vi "Valves_Combination.vi"   [LabVIEW 2011]
uses:
  Pumps_Valves_Dependencies_Global.vi
panel:
  # "Everything is in the block diagram.This vi updates the global combination booleans."
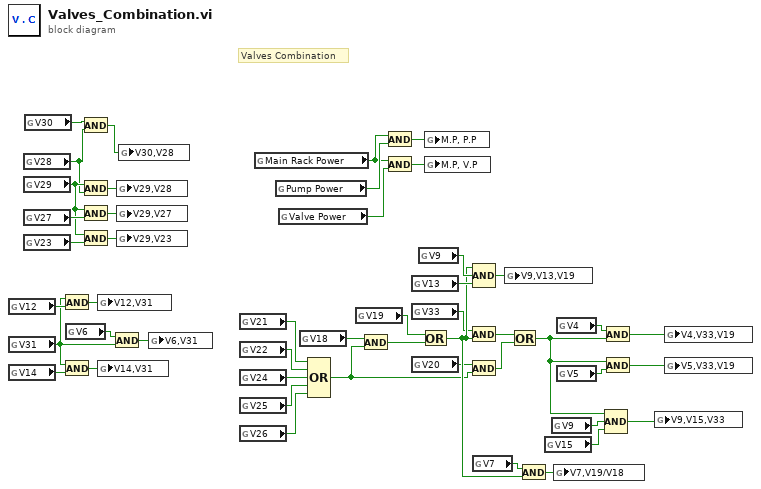
[diagram p0: block diagram]
diagram:
  # "Valves Combination"
  n1 = global read "Pumps_Valves_Dependencies_Global.vi" "V12"() -> (w30:bool)
  n2 = global read "Pumps_Valves_Dependencies_Global.vi" "V31"() -> (w29:bool)
  n3 = global read "Pumps_Valves_Dependencies_Global.vi" "V14"() -> (w31:bool)
  n4 = global read "Pumps_Valves_Dependencies_Global.vi" "V28"() -> (w1:bool)
  n5 = global read "Pumps_Valves_Dependencies_Global.vi" "V29"() -> (w46:bool)
  n6 = global read "Pumps_Valves_Dependencies_Global.vi" "V27"() -> (w48:bool)
  n7 = global read "Pumps_Valves_Dependencies_Global.vi" "V23"() -> (w47:bool)
  n8 = global read "Pumps_Valves_Dependencies_Global.vi" "V30"() -> (w2:bool)
  n9 = And(x=w29, y=w30) -> (x .and. y?=w25:bool)
  n10 = And(x=w29, y=w31) -> (x .and. y?=w24:bool)
  n11 = global read "Pumps_Valves_Dependencies_Global.vi" "V6"() -> (w32:bool)
  n12 = And(x=w2, y=w1) -> (x .and. y?=w3:bool)
  n13 = And(x=w46, y=w1) -> (x .and. y?=w18:bool)
  n14 = And(x=w46, y=w48) -> (x .and. y?=w19:bool)
  n15 = And(x=w46, y=w47) -> (x .and. y?=w20:bool)
  n16 = global write "Pumps_Valves_Dependencies_Global.vi" "V12,V31"(w25) -> ()
  n17 = global write "Pumps_Valves_Dependencies_Global.vi" "V14,V31"(w24) -> ()
  n18 = And(x=w32, y=w29) -> (x .and. y?=w23:bool)
  n19 = global write "Pumps_Valves_Dependencies_Global.vi" "V29,V28"(w18) -> ()
  n20 = global write "Pumps_Valves_Dependencies_Global.vi" "V29,V27"(w19) -> ()
  n21 = global write "Pumps_Valves_Dependencies_Global.vi" "V29,V23"(w20) -> ()
  n22 = global write "Pumps_Valves_Dependencies_Global.vi" "V30,V28"(w3) -> ()
  n23 = global write "Pumps_Valves_Dependencies_Global.vi" "V6,V31"(w23) -> ()
  n24 = global read "Pumps_Valves_Dependencies_Global.vi" "V21"() -> (w45:bool)
  n25 = global read "Pumps_Valves_Dependencies_Global.vi" "V22"() -> (w44:bool)
  n26 = global read "Pumps_Valves_Dependencies_Global.vi" "V24"() -> (w43:bool)
  n27 = global read "Pumps_Valves_Dependencies_Global.vi" "V25"() -> (w42:bool)
  n28 = global read "Pumps_Valves_Dependencies_Global.vi" "V26"() -> (w41:bool)
  n29 = global read "Pumps_Valves_Dependencies_Global.vi" "Main Rack Power"() -> (w26:bool)
  n30 = global read "Pumps_Valves_Dependencies_Global.vi" "Pump Power"() -> (w28:bool)
  n31 = global read "Pumps_Valves_Dependencies_Global.vi" "Valve Power"() -> (w27:bool)
  n32 = global read "Pumps_Valves_Dependencies_Global.vi" "V18"() -> (w40:bool)
  n33 = Compound Arithmetic op=OR(w45, w44, w43, w42, w41) -> (w8:bool)
  n34 = global read "Pumps_Valves_Dependencies_Global.vi" "V19"() -> (w39:bool)
  n35 = And(x=w40, y=w8) -> (x .and. y?=w38:bool)
  n36 = And(x=w26, y=w28) -> (x .and. y?=w22:bool)
  n37 = And(x=w26, y=w27) -> (x .and. y?=w21:bool)
  n38 = global read "Pumps_Valves_Dependencies_Global.vi" "V13"() -> (w35:bool)
  n39 = global read "Pumps_Valves_Dependencies_Global.vi" "V33"() -> (w12:bool)
  n40 = global read "Pumps_Valves_Dependencies_Global.vi" "V20"() -> (w13:bool)
  n41 = global read "Pumps_Valves_Dependencies_Global.vi" "V9"() -> (w34:bool)
  n42 = Or(x=w39, y=w38) -> (x .or. y?=w33:bool)
  n43 = global write "Pumps_Valves_Dependencies_Global.vi" "M.P, P.P"(w22) -> ()
  n44 = global write "Pumps_Valves_Dependencies_Global.vi" "M.P, V.P"(w21) -> ()
  n45 = And(x=w12, y=w33) -> (x .and. y?=w9:bool)
  n46 = And(x=w13, y=w8) -> (x .and. y?=w10:bool)
  n47 = Compound Arithmetic op=AND(w33, w34, w35) -> (w17:bool)
  n48 = global read "Pumps_Valves_Dependencies_Global.vi" "V7"() -> (w11:bool)
  n49 = global write "Pumps_Valves_Dependencies_Global.vi" "V9,V13,V19"(w17) -> ()
  n50 = Or(x=w9, y=w10) -> (x .or. y?=w6:bool)
  n51 = And(x=w11, y=w33) -> (x .and. y?=w14:bool)
  n52 = global read "Pumps_Valves_Dependencies_Global.vi" "V15"() -> (w4:bool)
  n53 = global read "Pumps_Valves_Dependencies_Global.vi" "V9"() -> (w5:bool)
  n54 = global write "Pumps_Valves_Dependencies_Global.vi" "V7,V19/V18"(w14) -> ()
  n55 = global read "Pumps_Valves_Dependencies_Global.vi" "V4"() -> (w37:bool)
  n56 = global read "Pumps_Valves_Dependencies_Global.vi" "V5"() -> (w36:bool)
  n57 = And(x=w37, y=w6) -> (x .and. y?=w16:bool)
  n58 = And(x=w6, y=w36) -> (x .and. y?=w15:bool)
  n59 = Compound Arithmetic op=AND(w6, w5, w4) -> (w7:bool)
  n60 = global write "Pumps_Valves_Dependencies_Global.vi" "V9,V15,V33"(w7) -> ()
  n61 = global write "Pumps_Valves_Dependencies_Global.vi" "V4,V33,V19"(w16) -> ()
  n62 = global write "Pumps_Valves_Dependencies_Global.vi" "V5,V33,V19"(w15) -> ()
